vi "trash-1.vi"   [LabVIEW 2014]
uses:
  <vilib>/Analysis/2dsp.llb/Integral Method.ctl
  <vilib>/Analysis/NI_AALPro.lvlib
  <vilib>/Analysis/8numeric.llb/1D Numeric Integration.vi
types:
  T1 = typedef "NI_AALPro.lvlib/Integral Method.ctl" = i32
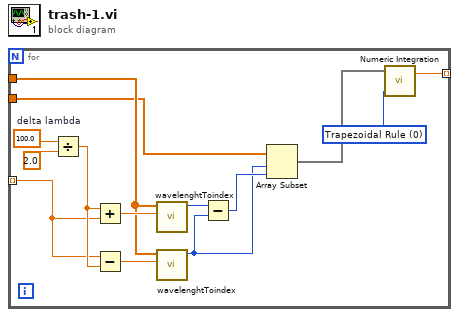
[diagram p0: block diagram]
diagram:
  n1 = for {
    tunnel: _ -> [w11] mode=indexing
    tunnel: _ -> [w8]
    tunnel: _ -> [w6]
    tunnel: [w2] -> _ mode=indexing
    w3 = T1 0 items=["Trapezoidal Rule", "Simpson's Rule", "Simpson's 3/8 Rule", "Bode Rule"] ("integration method")
    w14 = 100.0  # delta lambda
    n2 = Divide(x=w14, y=2.0) -> (x/y=w12:dbl)
    n3 = Add(x=w12, y=w11) -> (x+y=w10:dbl)
    n4 = Subtract(x=w11, y=w12) -> (x-y=w9:dbl)
    n5 = call "wavelenghtToindex.vi"("WL in"=w10, "WL Values"=w8) -> ("index of WL"=w7:i32)  [unwired: 9 in]
    n6 = call "wavelenghtToindex.vi"("WL in"=w9, "WL Values"=w8) -> ("index of WL"=w4:i32)  [unwired: 9 in]
    n7 = Subtract(x=w7, y=w4) -> (x-y=w5:i32)
    n8 = Array Subset(array=w6, index=w4, length=w5) -> (w1:void[])
    n9 = call-poly <vilib>:"Numeric Integration.vi"("integration method"=w3, "Input Array"=w1) -> ("result"=w2:dbl)  [unwired: 1 in, 1 out]
  }
